vi "TCP.IP Client for Ripple Detection_maybe2.vi"() -> ()   [LabVIEW 2021]
doc: "Demonstrates how to open a connection to an TCP server, read the data being sent, and display the data on a chart. This VI is designed to stop if the TCP connection is terminated."
uses:
  <vilib>/Analysis/3filter.llb/Butterworth Filter (DBL).vi
  <vilib>/ptbypt/NI_PtbyPt.lvlib
  <vilib>/Analysis/NI_AALBase.lvlib
panel:
  in  "File Name":path=path "F:/Career/Work/From Now/Book2.csv"
  out "Filtered":dbl[](graph)
  out "Array Size 3":u32
  out "Delayed RMS2>RMS1 for 3 data":dynamicdata(graph)
  out "RMS2>RMS1 for 3 data":dynamicdata(graph)
  out "Array Size":u32
  out "RMS2>RMS1":dynamicdata(graph)
  out "RMS1":dynamicdata(graph)
  out "RMS2":dynamicdata(graph)
  out "Raw Data Collected":dynamicdata(graph)
  in  "Boolean":bool
  in  "Server Closed":string="The server VI closed the connection."
  out "Raw Data":dbl[](graph)
  in  "Stop":bool
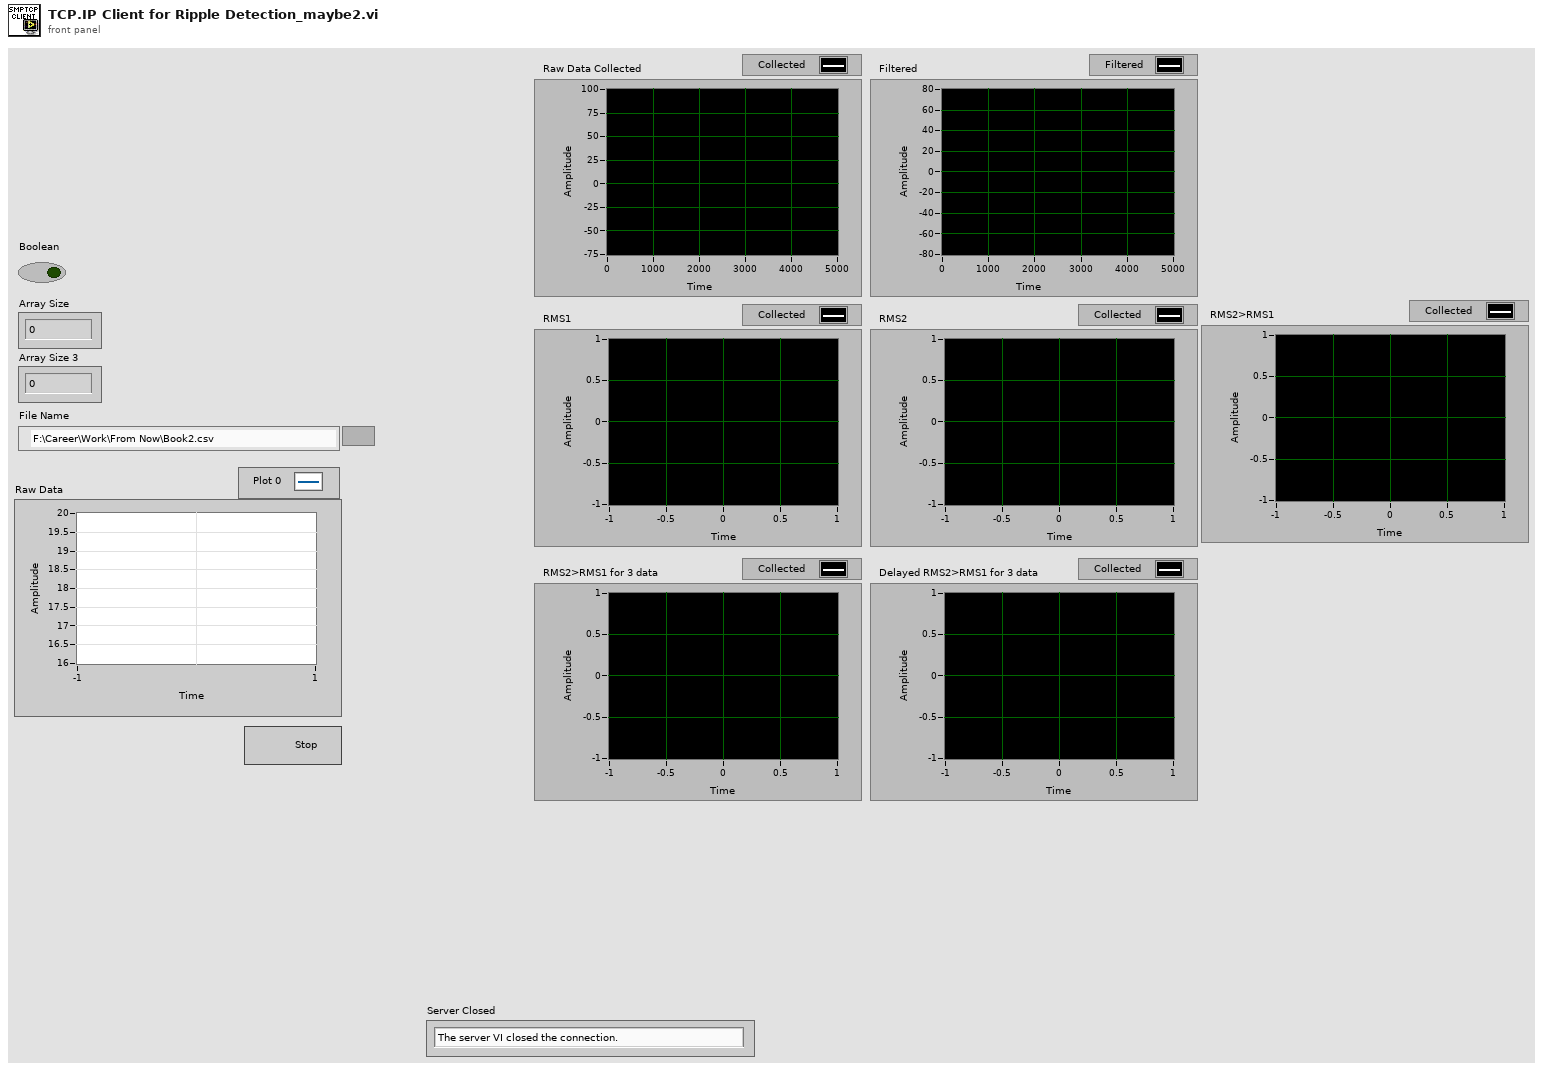
[diagram p1: front panel]
types:
  T1 = enum16{"open", "replace", "create", "open or create", "replace or create", "replace or create with confirmation"}
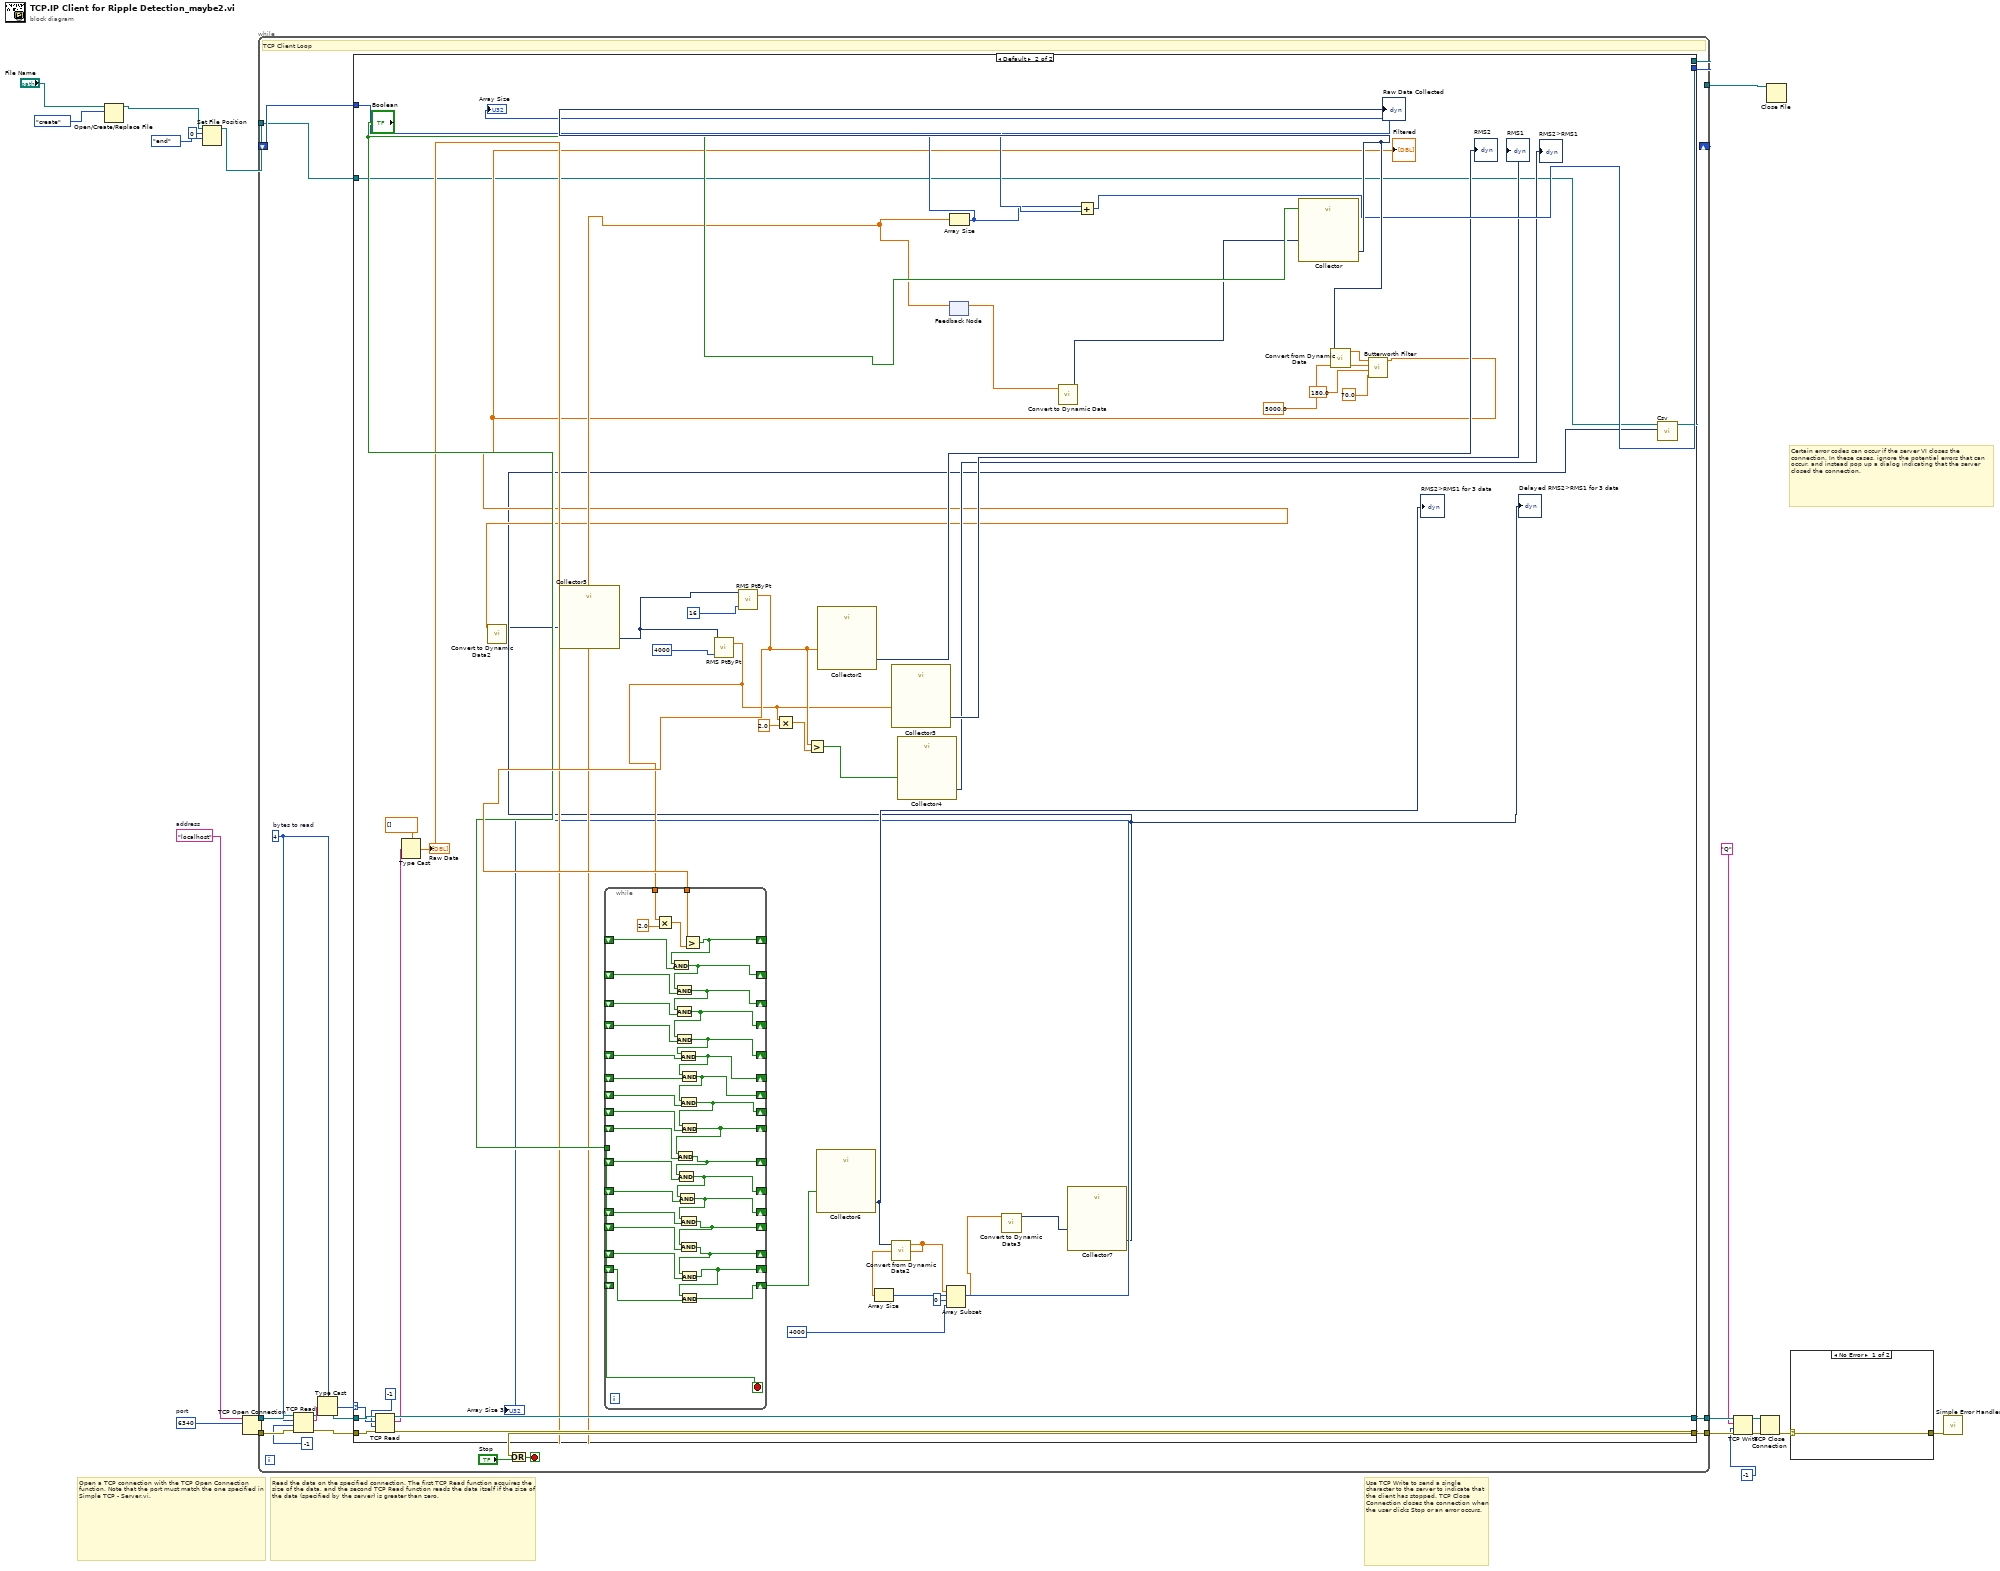
[diagram p0: block diagram]
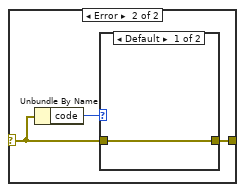
[diagram p2: hidden frame]
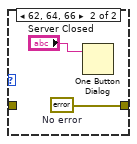
[diagram p3: hidden frame]
diagram:
  w9 = u16 6340  # port
  w10 = "localhost"  # address
  # "Certain error codes can occur if the server VI closes the connection. In these cases, ignore the potential errors that can occur, and instead pop up a dialog indicating that the server closed the connection."
  # "Use TCP Write to send a single character to the server to indicate that the client has stopped. TCP Close Connection closes the connection when the user clicks Stop or an error occurs."
  # "Read the data on the specified connection. The first TCP Read function acquires the size of the data, and the second TCP Read function reads the data itself if the size of the data (specified by the server) is greater than zero."
  # "Open a TCP connection with the TCP Open Connection function. Note that the port must match the one specified in Simple TCP - Server.vi."
  n1 = Open/Create/Replace File(file path (use dialog)="File Name", operation (0:open)=T1."create") -> (refnum out=w3:refnum<file>)  [unwired: 4 in, 2 out]
  n2 = Set File Position(offset (in bytes) (0)=i64 0, refnum=w3, from (0:start)=enum16{"start", "end", "current"}."end") -> (refnum out=w2:refnum<file>)  [unwired: 1 in, 1 out]
  n3 = TCP Open Connection(address=w10, remote port or service name=w9) -> (connection ID=w19:refnum<k5>, error out=w18:errorcluster)  [unwired: 3 in]
  n4 = while {
    tunnel: w18 -> [w31]
    tunnel: w19 -> [w32]
    tunnel: [w27] -> w16
    tunnel: [w26] -> w14
    shift-right: [w22] -> _
    shift-left: _ -> [w23]
    tunnel: [w21] -> w8
    tunnel: w2 -> [w20]
    stop <- w28 stop-if-true
    w30 = 4  # bytes to read
    # "TCP Client Loop"
    n5 = TCP Read(connection ID=w32, bytes to read=w30, error in (no error)=w31, 9:-1 ("timeout ms (25000)")) -> (connection ID out=w34:refnum<k5>, data out=w35:string, error out=w33:errorcluster)  [unwired: 1 in]
    n6 = Type Cast(type=w30, x=w35) -> (*(type *) &x=w25:i32)
    n7 = case shown="Default" w25 {
      selector: w25 -> [_ w77]
      tunnel: w34 -> [w39 w83]
      tunnel: w33 -> [w38 w82]
      tunnel: [w39 w80] -> w27
      tunnel: [w38 w79] -> w26
      tunnel: w23 -> [w37 w72]
      tunnel: [w37 w71] -> w22
      tunnel: w20 -> [w36 w61]
      tunnel: [w36 w60] -> w21
      frame ..0 {
        # "The server has not written any data"
      }
      frame Default {
        n8 = TCP Read(connection ID=w83, bytes to read=w77, error in (no error)=w82, 9:-1 ("timeout ms (25000)")) -> (connection ID out=w80:refnum<k5>, data out=w78:string, error out=w79:errorcluster)  [unwired: 1 in]
        n9 = Type Cast(type=dbl[] [] ("chart"), x=w78) -> (*(type *) &x=w70:dbl[])
        "Raw Data" <- w70
        n10 = feedback #1() -> (w54:dbl[])  [unwired: 1 in]
        n11 = feedback-in #1(w70) -> ()
        n12 = Array Size(array=w70) -> (size(s)=w69:i32)
        "Array Size" <- w69
        n13 = call "Convert to Dynamic Data"("Array"=w54) -> ("Dynamic Data Type"=w55:dynamicdata)  [unwired: 3 in]
        n14 = Add(x=w69, y=w72) -> (x+y=w71:i32)
        n15 = call "Collector"("Enable"="Boolean", "Signals"=w55) -> ("Collected Signals"=w76:dynamicdata)  [unwired: 8 in, 1 out]
        "Raw Data Collected" <- w76
        n16 = call "Convert from Dynamic Data"("Dynamic Data Type"=w76) -> ("Array"=w56:dbl[])  [unwired: 3 in]
        n17 = call-poly <vilib>:"Butterworth Filter.vi"("low cutoff freq: fl"=70.0, "high cutoff freq: fh"=180.0, "sampling freq: fs"=5000.0, "X"=w56) -> ("Filtered X"=w63:dbl[])  [unwired: 4 in, 1 out]
        "Filtered" <- w63
        n18 = call "Convert to Dynamic Data2"("Array"=w63) -> ("Dynamic Data Type"=w48:dynamicdata)  [unwired: 3 in]
        n19 = call "Collector5"("Signals"=w48) -> ("Collected Signals"=w47:dynamicdata)  [unwired: 9 in, 1 out]
        n20 = call <vilib>:"RMS PtByPt.vi"("sample length"=4000, "x"=w47) -> ("rms value"=w74:dbl)  [unwired: 2 in, 1 out]
        n21 = call <vilib>:"RMS PtByPt.vi"("sample length"=16, "x"=w47) -> ("rms value"=w75:dbl)  [unwired: 2 in, 1 out]
        n22 = while {
          tunnel: w75 -> [w117]
          tunnel: w74 -> [w116]
          shift-right: [w111] -> _
          shift-left: _ -> [w112]
          shift-right: [w114] -> _
          shift-left: _ -> [w113]
          tunnel: "Boolean" -> [w115]
          shift-right: [w109] -> _
          shift-left: _ -> [w110]
          shift-right: [w107] -> _
          shift-left: _ -> [w108]
          shift-right: [w106] -> _
          shift-left: _ -> [w105]
          shift-right: [w97] -> _
          shift-left: _ -> [w90]
          shift-right: [w102] -> _
          shift-left: _ -> [w101]
          shift-right: [w104] -> _
          shift-left: _ -> [w103]
          shift-right: [w99] -> _
          shift-left: _ -> [w100]
          shift-right: [w98] -> _
          shift-left: _ -> [w91]
          shift-right: [w96] -> _
          shift-left: _ -> [w89]
          shift-right: [w95] -> _
          shift-left: _ -> [w88]
          shift-right: [w94] -> _
          shift-left: _ -> [w87]
          shift-right: [w93] -> _
          shift-left: _ -> [w86]
          shift-right: [w92] -> _
          shift-left: _ -> [w85]
          shift-right: [w84] -> w41
          shift-left: _ -> [_]
          stop <- w115 stop-if-true
          n23 = Multiply(x=w116, y=2.0) -> (x*y=w118:dbl)
          n24 = Greater?(x=w117, y=w118) -> (0:w114:bool)
          n25 = And(x=w114, y=w113) -> (x .and. y?=w111:bool)
          n26 = And(x=w111, y=w112) -> (x .and. y?=w109:bool)
          n27 = And(x=w109, y=w110) -> (x .and. y?=w107:bool)
          n28 = And(x=w107, y=w108) -> (x .and. y?=w106:bool)
          n29 = And(x=w106, y=w105) -> (x .and. y?=w104:bool)
          n30 = And(x=w104, y=w103) -> (x .and. y?=w102:bool)
          n31 = And(x=w102, y=w101) -> (x .and. y?=w99:bool)
          n32 = And(x=w99, y=w100) -> (x .and. y?=w98:bool)
          n33 = And(x=w98, y=w91) -> (x .and. y?=w97:bool)
          n34 = And(x=w97, y=w90) -> (x .and. y?=w96:bool)
          n35 = And(x=w96, y=w89) -> (x .and. y?=w95:bool)
          n36 = And(x=w95, y=w88) -> (x .and. y?=w94:bool)
          n37 = And(x=w94, y=w87) -> (x .and. y?=w93:bool)
          n38 = And(x=w93, y=w86) -> (x .and. y?=w92:bool)
          n39 = And(x=w92, y=w85) -> (x .and. y?=w84:bool)
        }
        n40 = Multiply(x=w74, y=2.0) -> (x*y=w50:dbl)
        n41 = Greater?(x=w75, y=w50) -> (0:w49:bool)
        n42 = call "Collector6"("Signals"=w41) -> ("Collected Signals"=w65:dynamicdata)  [unwired: 9 in, 1 out]
        "RMS2>RMS1 for 3 data" <- w65
        n43 = call "Collector2"("Signals"=w75) -> ("Collected Signals"=→"RMS2":dynamicdata)  [unwired: 9 in, 1 out]
        n44 = call "Collector3"("Signals"=w74) -> ("Collected Signals"=→"RMS1":dynamicdata)  [unwired: 9 in, 1 out]
        n45 = call "Convert from Dynamic Data2"("Dynamic Data Type"=w65) -> ("Array"=w43:dbl[])  [unwired: 3 in]
        n46 = Array Size(array=w43) -> (size(s)=→"Array Size 3":i32)
        n47 = call "Collector4"("Signals"=w49) -> ("Collected Signals"=→"RMS2>RMS1":dynamicdata)  [unwired: 9 in, 1 out]
        n48 = Array Subset(array=w43, index=0, length=4000 ("index")) -> (w42:dbl[])
        n49 = call "Convert to Dynamic Data3"("Array"=w42) -> ("Dynamic Data Type"=w46:dynamicdata)  [unwired: 3 in]
        n50 = call "Collector7"("Signals"=w46) -> ("Collected Signals"=w62:dynamicdata)  [unwired: 9 in, 1 out]
        "Delayed RMS2>RMS1 for 3 data" <- w62
        n51 = call "Csv.vi"("Delayed RMS2>RMS1 for 3 data"=w62, "Byte Stream File in"=w61) -> ("Byte Stream File out"=w60:refnum<file>)  [unwired: 9 in]
      }
    }
    n52 = Or(x=w26, y="Stop") -> (x .or. y?=w28:bool)
  }
  n53 = TCP Write(connection ID=w16, data in="Q", error in (no error)=w14, 9:-1 ("timeout ms (25000)")) -> (connection ID out=w17:refnum<k5>, error out=w15:errorcluster)  [unwired: 1 out]
  n54 = TCP Close Connection(connection ID=w17, error in (no error)=w15) -> (error out=w12:errorcluster)  [unwired: 1 in, 1 out]
  n55 = Close File(refnum=w8) -> ()  [unwired: 1 in, 2 out]
  n56 = case shown="No Error" w12 {
    selector: w12 -> [w120 w122]
    tunnel: [w120 w121] -> w11
    frame No Error {
    }
    frame Error {
      n57 = Unbundle By Name(w122) -> ("code"=w123:i32)
      n58 = case shown="Default" w123 {
        tunnel: w122 -> [w124 _]
        tunnel: [w124 w126] -> w121
        frame Default {
        }
        frame 62, 64, 66 {
          w126 = errorcluster {"status"=FALSE, "code"=0, "source"=""}  # No error
          n59 = One Button Dialog(message="Server Closed") -> ()  [unwired: 1 in, 1 out]
        }
      }
    }
  }
  n60 = call <vilib>:"Simple Error Handler.vi"("error in (no error)"=w11) -> ()  [unwired: 4 in, 5 out]
